vi "Get 湿度.vi"(11 "THM-V6数字型温湿度 in":refnum<class "THM-V6数字型温湿度.lvclass">) -> (2 "湿度":refnum<vi>, 3 "THM-V6数字型温湿度 out":refnum<class "THM-V6数字型温湿度.lvclass">)   [LabVIEW 2016, in "THM-V6数字型温湿度.lvlib" / "THM-V6数字型温湿度.lvclass"]
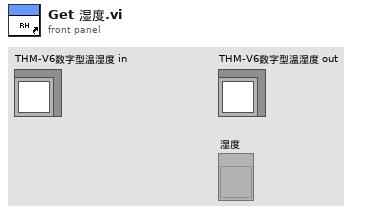
[diagram p1: front panel]
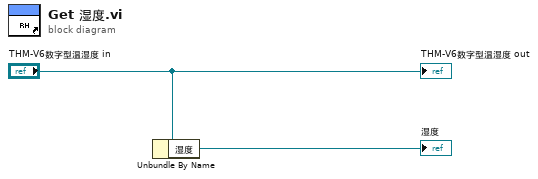
[diagram p0: block diagram]
diagram:
  n1 = Unbundle By Name("THM-V6数字型温湿度 in") -> ("湿度"=→"湿度":refnum<vi>)
  "THM-V6数字型温湿度 out" <- "THM-V6数字型温湿度 in"
